vi "fix class control labels.vi"(8 "error in":errorcluster, 10 "class to load":path, 11 "application in":refnum<vi>) -> (0 "error out":errorcluster)   [LabVIEW 2014, in "SequencerActionScript.lvclass"]
doc: "NI Tag Bus Module Framework 1.0.2.36\nNI Systems Engineering"
uses:
  SequencerActionScript.lvclass
  <vilib>/Utility/traverseref.llb/TRef TravTarget.ctl
  <vilib>/Utility/traverseref.llb/VI Scripting - Traverse.lvlib
  <vilib>/Utility/VariantDataType/VariantType.lvlib
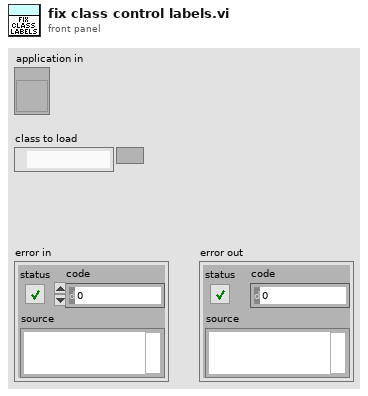
[diagram p1: front panel]
types:
  T1 = typedef "TRef TravTarget.ctl" = enum16{"FP", "BD", "Other"}
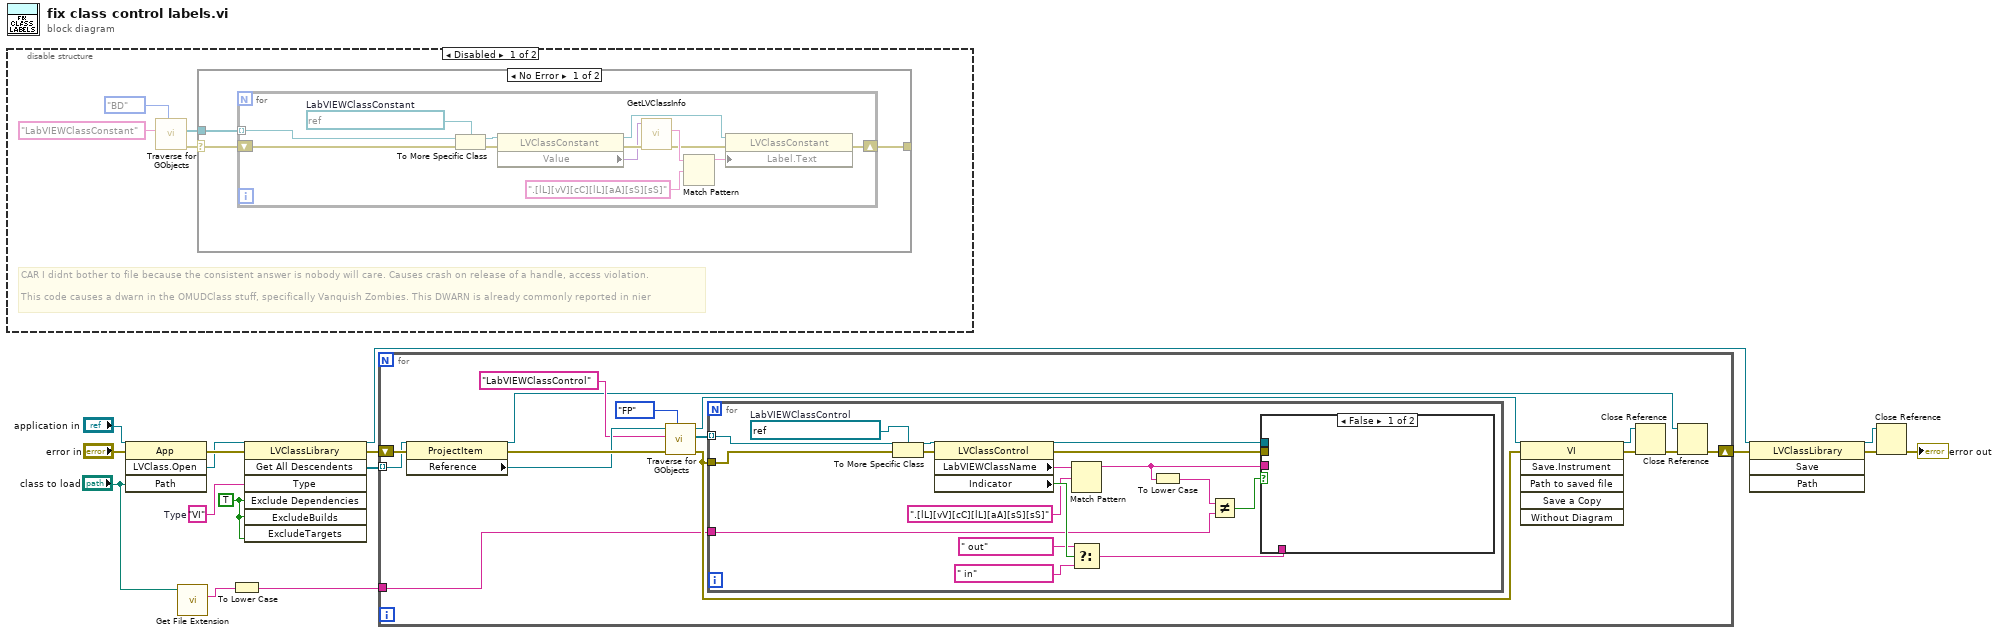
[diagram p0: block diagram]
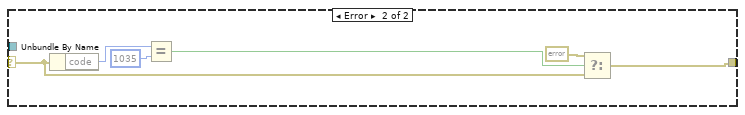
[diagram p2: hidden frame]
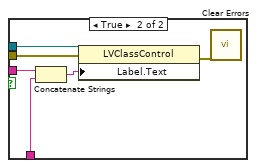
[diagram p4: hidden frame]
diagram:
  w12 = TRUE
  w11 = "VI"  # Type
  n1 = disable-structure shown="Disabled" {
    frame Disabled {
      # "CAR I didnt bother to file because the consistent answer is nobody will care. Causes crash on release of a handle, access violation. \n\nThis code causes a dwarn in the OMUDClass stuff, specifically Vanquish Zombies. This DWARN is already commonly reported in nier"
      n2 = call <vilib>:"Traverse for GObjects.vi"("Traverse Target"=TRef_TravTarget."BD", "Class Name"="LabVIEWClassConstant") -> ("error out"=w22:errorcluster, "References"=w21:refnum<vi>[], "dup VI Refnum"=w23:refnum<vi>, "error in (no error)"=w19:errorcluster, "VI Refnum"=w20:refnum<vi>)  [unwired: 4 in, 1 out]
      n3 = case shown="No Error" w22 {
        selector: w22 -> [w24 w42]
        tunnel: [w26 w40] -> _
        tunnel: w21 -> [w25 _]
        frame No Error {
          n4 = for {
            shift-right: [w34] -> w26
            shift-left: w24 -> [w39]
            tunnel: w25 -> [w37] mode=indexing
            w33 = refnum<vi> refnum  # LabVIEWClassConstant
            n5 = To More Specific Class(target class=w33, reference=w37, error in=w39) -> (specific class reference=w36:refnum<vi>, error out=w38:errorcluster)
            n6 = property class="LVClassConstant"(reference=w36, error in=w38) -> (reference out=w35:refnum<vi>, error out=w30:errorcluster, "Value"=w29:variant)
            n7 = call <vilib>:"GetLVClassInfo.vi"("error in (no error)"=w30, "Variant"=w29) -> ("error out"=w27:errorcluster, "LV Class File Name"=w28:string)  [unwired: 7 in, 1 out]
            n8 = Match Pattern(string=w28, regular expression=".[lL][vV][cC][lL][aA][sS][sS]") -> (before substring=w31:string)  [unwired: 1 in, 3 out]
            n9 = property class="LVClassConstant"(reference=w35, error in=w27, "Label.Text"=w31) -> (error out=w34:errorcluster)  [unwired: 1 out]
          }
        }
        frame Error {
          n10 = Unbundle By Name(w42) -> ("code"=w45:i32)
          n11 = Equal?(x=w45, y=1035) -> (x = y?=w43:bool)
          n12 = Select(t=errorcluster {"status"=FALSE, "code"=0, "source"=""}, s=w43, f=w42) -> (s? t:f=w40:errorcluster)
        }
      }
    }
    frame Enabled {
    }
  }
  n13 = invoke class="App" method="LVClass.Open"(reference="application in", error in="error in", "Path"="class to load") -> (error out=w13:errorcluster, "LVClass.Open"=w10:refnum<vi>)  [unwired: 1 in, 2 out]
  n14 = call <vilib>:"Get File Extension.vi"("file"="class to load") -> ("lowercase file extension"=w2:string)  [unwired: 7 in, 3 out]
  n15 = To Lower Case(string=w2) -> (all lower case string=w1:string)
  n16 = invoke class="LVClassLibrary" method="Get All Descendents"(reference=w10, error in=w13, "Type"=w11, "Exclude Dependencies"=w12, "ExcludeBuilds"=w12, "ExcludeTargets"=w12) -> (reference out=w8:refnum<vi>, error out=w15:errorcluster, "All Descendents"=w14:refnum<vi>[])  [unwired: 1 in, 4 out]
  n17 = for {
    tunnel: w14 -> [w59] mode=indexing
    shift-right: [w51] -> w16
    shift-left: w15 -> [w60]
    tunnel: w1 -> [w46]
    n18 = property class="ProjectItem"(reference=w59, error in=w60) -> (reference out=w50:refnum<vi>, error out=w58:errorcluster, "Reference"=w57:refnum<vi>)
    n19 = call <vilib>:"Traverse for GObjects.vi"("Traverse Target"=TRef_TravTarget."FP", "error in (no error)"=w58, "Class Name"="LabVIEWClassControl", "VI Refnum"=w57) -> ("error out"=w47:errorcluster, "References"=w54:refnum<vi>[], "dup VI Refnum"=w53:refnum<vi>)  [unwired: 4 in, 1 out]
    n20 = for {
      tunnel: w54 -> [w76] mode=indexing
      tunnel: w47 -> [w65]
      tunnel: w46 -> [w62]
      w74 = refnum<vi> refnum  # LabVIEWClassControl
      n21 = To More Specific Class(target class=w74, reference=w76, error in=w65) -> (specific class reference=w75:refnum<vi>, error out=w77:errorcluster)
      n22 = property class="LVClassControl"(reference=w75, error in=w77) -> (reference out=w73:refnum<vi>, error out=w72:errorcluster, "LabVIEWClassName"=w67:string, "Indicator"=w71:bool)
      n23 = Match Pattern(string=w67, regular expression=".[lL][vV][cC][lL][aA][sS][sS]") -> (before substring=w64:string)  [unwired: 1 in, 3 out]
      n24 = Select(t=" out", s=w71, f=" in") -> (s? t:f=w68:string)
      n25 = To Lower Case(string=w64) -> (all lower case string=w63:string)
      n26 = Not Equal?(x=w63, y=w62) -> (x != y?=w61:bool)
      n27 = case shown="False" w61 {
        tunnel: w73 -> [_ w83]
        tunnel: w72 -> [_ w82]
        tunnel: w68 -> [_ w80]
        tunnel: w64 -> [_ w78]
        frame False {
        }
        frame True {
          n28 = Concatenate Strings(w78, w80) -> (w81:string)
          n29 = property class="LVClassControl"(reference=w83, error in=w82, "Label.Text"=w81) -> (error out=w79:errorcluster)  [unwired: 1 out]
          n30 = call <vilib>:"Clear Errors.vi"("error in (no error)"=w79) -> ()  [unwired: 5 in, 2 out]
        }
      }
    }
    n31 = invoke class="VI" method="Save.Instrument"(reference=w53, error in=w47) -> (reference out=w48:refnum<vi>, error out=w49:errorcluster)  [unwired: 4 in, 4 out]
    n32 = Close Reference(reference=w48, error in (no error)=w49) -> (error out=w52:errorcluster)
    n33 = Close Reference(reference=w50, error in (no error)=w52) -> (error out=w51:errorcluster)
  }
  n34 = invoke class="LVClassLibrary" method="Save"(reference=w8, error in=w16) -> (reference out=w7:refnum<vi>, error out=w9:errorcluster)  [unwired: 2 in, 2 out]
  n35 = Close Reference(reference=w7, error in (no error)=w9) -> (error out=→"error out":errorcluster)
